vi "Pixel integration - Pulse width.vi"(8 "error in (no error)":errorcluster, 10 "channel":i32, 11 "tagger in":refnum<k24>) -> (0 "error out":errorcluster, 1 "pixel_end_ch":i32, 2 "pixel_start_ch":i32)   [LabVIEW 2014]
uses:
  SwabianInstruments.TimeTagger
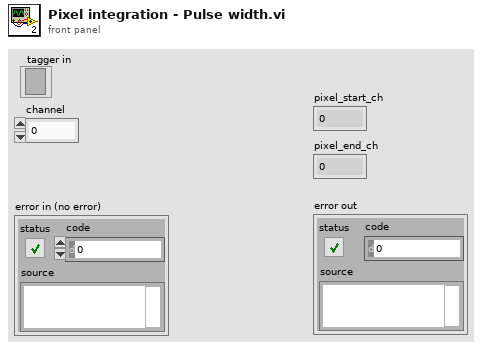
[diagram p1: front panel]
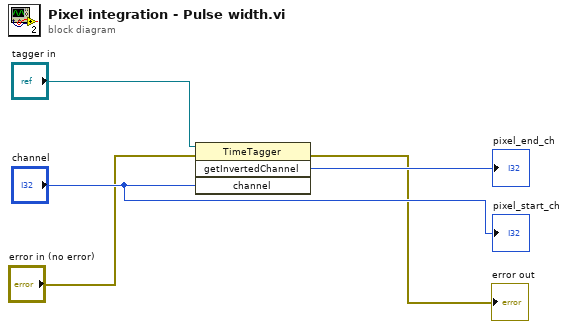
[diagram p0: block diagram]
diagram:
  n1 = invoke class="TimeTagger" method="getInvertedChannel"(reference="tagger in", error in="error in (no error)", "channel"="channel") -> (error out=→"error out":errorcluster, "getInvertedChannel"=→"pixel_end_ch":i32)  [unwired: 1 in, 2 out]
  "pixel_start_ch" <- "channel"
